vi "chceksystem.vi"(8 "error in (no error)":errorcluster, 10 "Required software":string[](array[string])=["NI Vision Common Resources 2016", "NI-VISA 16.0", "NI-VISA Configuration Support 16.0", "NI-VISA Runtime 16.0", "NI Vision 2016", "NI Vision Runtime 2016", "NI LabVIEW Unit Test Framework Toolkit", "NI LabVIEW VI Analyzer Toolkit", "NI-IMAQdx 16.0", "NI-IMAQdx Runtime 16.0"]) -> (0 "Error out":errorcluster, 1 "OK?":bool, 2 "Array":string[](array[string]))   [LabVIEW 2016]
uses:
  <vilib>/nisyscfg/Software 1.2.ctl
  <vilib>/nisyscfg/Component Type.ctl
  <vilib>/nisyscfg/Get Installed Components.vi
  <vilib>/Utility/error.llb/Error Cluster From Error Code.vi
  <vilib>/ErrorRing/Error Ring.xnode
  <vilib>/nisyscfg/nisyscfg.lvlib
panel:
  out "Software Components":T1[](array[typedef]) {"component type" items=["standard", "hidden", "system", "unknown", "startup", "image"]}
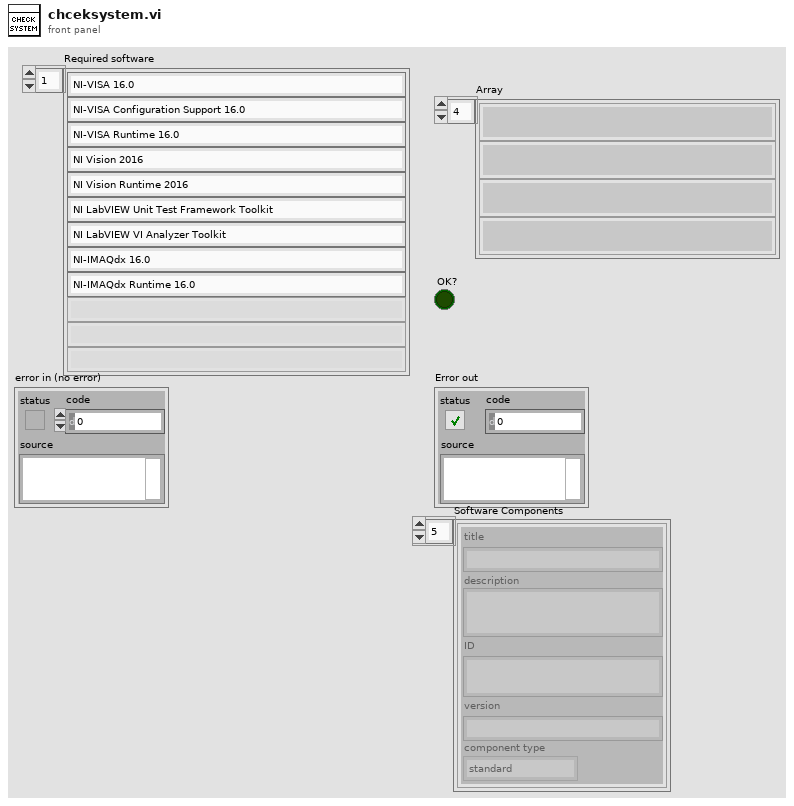
[diagram p1: front panel]
types:
  T1 = typedef "nisyscfg.lvlib/Software 1.2.ctl" = cluster{"title":string, "description":string, "ID":string, "version":string, "component type":T2}
  T2 = typedef "nisyscfg.lvlib/Component Type.ctl" = u32
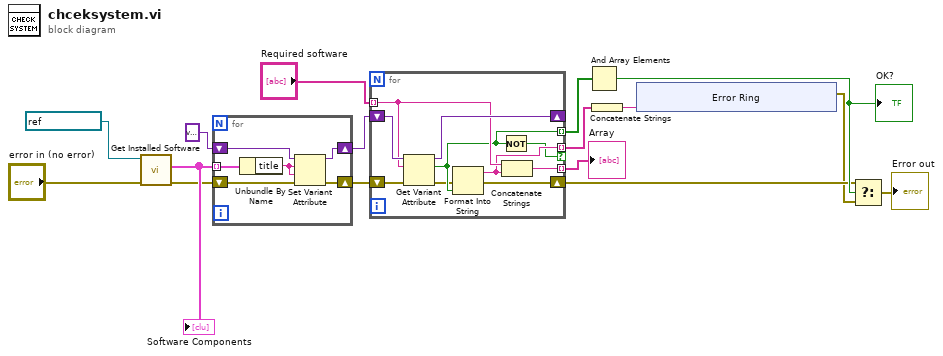
[diagram p0: block diagram]
diagram:
  n1 = call-poly <vilib>:"Get Installed Software.vi"("error in (no error)"="error in (no error)", "Session in"=refnum<k21> "localhost") -> ("error out"=w13:errorcluster, "Software Components"=w15:T1[])  [unwired: 7 in, 1 out]
  "Software Components" <- w15
  n2 = for {
    tunnel: w15 -> [w22] mode=indexing
    shift-right: [w20] -> w11
    shift-left: variant -> [w21]
    shift-right: [w18] -> w12
    shift-left: w13 -> [w19]
    n3 = Unbundle By Name(w22) -> ("title"=w17:string)
    n4 = Set Variant Attribute(Variant=w21, name=w17, value=w17, error in=w19) -> (Variant out=w20:variant, error out=w18:errorcluster)  [unwired: 1 out]
  }
  n5 = for {
    shift-right: [w30] -> _
    shift-left: w11 -> [w31]
    tunnel: "Required software" -> [w29] mode=indexing
    shift-right: [w23] -> w7
    shift-left: w12 -> [w32]
    tunnel: [w28] -> w2 mode=indexing
    tunnel: [w26] -> w9 mode=indexing
    tunnel: [w27] -> w5 mode=indexing if=w25
    n6 = Get Variant Attribute(Variant=w31, name=w29, error in=w32) -> (duplicate Variant=w30:variant, found=w26:bool, error out=w24:errorcluster)  [unwired: 1 in, 1 out]
    n7 = Format Into String(error in=w24, w26) -> (resulting string=w27:string, error out=w23:errorcluster)  [unwired: 2 in]
    n8 = Not(x=w26) -> (.not. x?=w25:bool)
    n9 = Concatenate Strings(w29, w27) -> (w28:string)
  }
  "Array" <- w2
  n10 = And Array Elements(Boolean array=w9) -> (logical AND=w8:bool)
  "OK?" <- w8
  n11 = Concatenate Strings(w5) -> (w4:string)
  n12 = xnode "Error Ring"("parameter 0"=w4) -> ("error out"=w6:errorcluster)
  n13 = Select(t=w7, s=w8, f=w6) -> (s? t:f=→"Error out":errorcluster)
